vi "Format_Request.vi"(8 "error in (no error)":errorcluster, 10 "Request":T1(ring), 11 "Request in":refnum<class "Request.lvclass">) -> (0 "error out":errorcluster, 3 "Request out":refnum<class "Request.lvclass">)   [LabVIEW 2016, in "Request.lvclass"]
uses:
  Request.lvclass
  Request.lvclass/Request.ctl
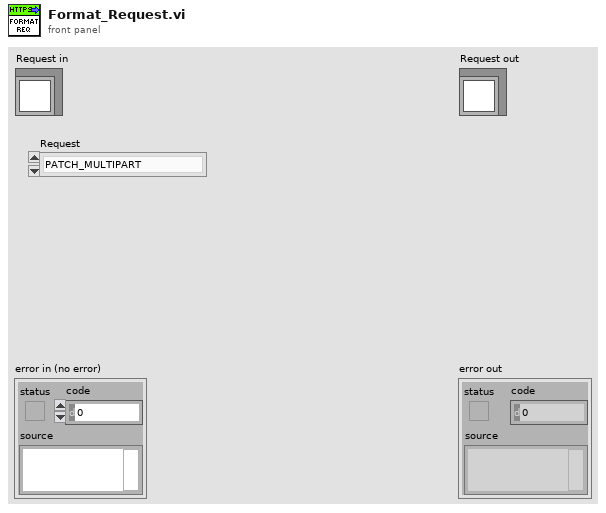
[diagram p1: front panel]
types:
  T1 = enum16{"PATCH_MULTIPART", "POST_MULTIPART", "PATCH", "DELETE", "HEAD", "PUT", "GET"}
  T2 = cluster{"Name":string, "Value":string, "File":path, "Filename":string, "MIME type":string}[]
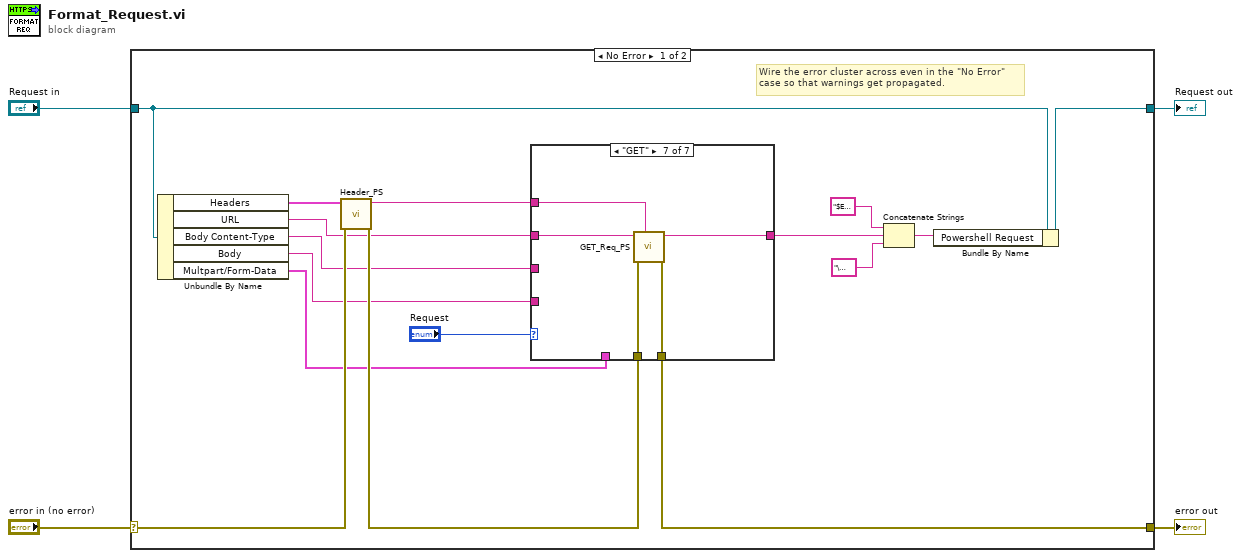
[diagram p0: block diagram]
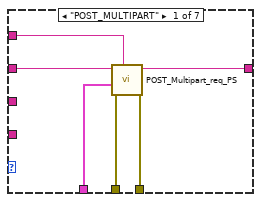
[diagram p2: hidden frame]
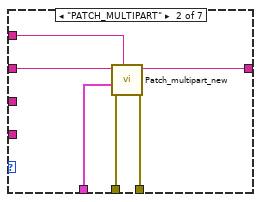
[diagram p3: hidden frame]
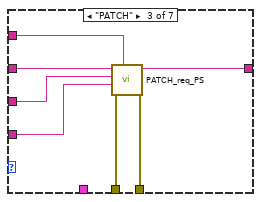
[diagram p4: hidden frame]
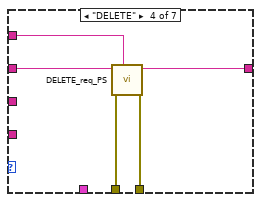
[diagram p5: hidden frame]
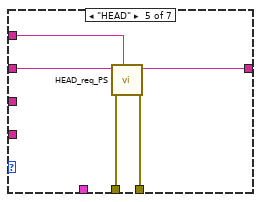
[diagram p6: hidden frame]
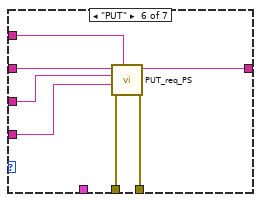
[diagram p7: hidden frame]
diagram:
  n1 = case shown="No Error" "error in (no error)" {
    selector: "error in (no error)" -> [w15 w63]
    tunnel: [w9 w63] -> w3
    tunnel: [w7 w62] -> w1
    tunnel: "Request in" -> [w8 w62]
    frame No Error {
      # "Wire the error cluster across even in the \"No Error\"\ncase so that warnings get propagated."
      n2 = Unbundle By Name(w8) -> ("Headers"=w14:cluster{"Name":string, "Value":string}[], "URL"=w13:string, "Body Content-Type"=w12:string, "Body"=w11:string, "Multpart/Form-Data"=w10:T2)
      n3 = call "Header_PS.vi"("error in"=w15, "Headers In"=w14) -> ("error out"=w16:errorcluster, "Headers_PS_Dict"=w17:string)  [unwired: 8 in]
      n4 = case shown="\"GET\"" "Request" {
        tunnel: w10 -> [w26 w27 _ _ _ _ _]
        tunnel: w13 -> [w23 w31 w39 w41 w47 w56 w58]
        tunnel: w16 -> [w25 w29 w38 w44 w49 w53 w59]
        tunnel: [w24 w28 w37 w43 w48 w52 w60] -> w9
        tunnel: w17 -> [w22 w32 w36 w40 w46 w51 w57]
        tunnel: [w21 w30 w33 w42 w45 w50 w61] -> w18
        tunnel: w12 -> [_ _ w34 _ _ w55 _]
        tunnel: w11 -> [_ _ w35 _ _ w54 _]
        frame "POST_MULTIPART" {
          n5 = call "POST_Multipart_req_PS.vi"("Headers"=w22, "error in"=w25, "Multpart/Form-Data"=w26, "URL"=w23) -> ("error out"=w24:errorcluster, "Multipart PATCH Request"=w21:string)  [unwired: 6 in]
        }
        frame "PATCH_MULTIPART" {
          n6 = call "Patch_multipart_new.vi"("Headers"=w32, "error in"=w29, "Multpart/Form-Data"=w27, "URL"=w31) -> ("error out"=w28:errorcluster, "Multipart PATCH Request"=w30:string)  [unwired: 6 in]
        }
        frame "PATCH" {
          n7 = call "PATCH_req_PS.vi"("Headers"=w36, "error in"=w38, "Body"=w35, "ContentType"=w34, "URL"=w39) -> ("error out"=w37:errorcluster, "PATCH Request"=w33:string)  [unwired: 5 in]
        }
        frame "DELETE" {
          n8 = call "DELETE_req_PS.vi"("Headers"=w40, "error in"=w44, "URL"=w41) -> ("error out"=w43:errorcluster, "DELETE Request"=w42:string)  [unwired: 7 in]
        }
        frame "HEAD" {
          n9 = call "HEAD_req_PS.vi"("Headers"=w46, "error in"=w49, "URL"=w47) -> ("error out"=w48:errorcluster, "HEAD Request"=w45:string)  [unwired: 7 in]
        }
        frame "PUT" {
          n10 = call "PUT_req_PS.vi"("Headers"=w51, "error in"=w53, "ContentType"=w54, "Body"=w55, "URL"=w56) -> ("error out"=w52:errorcluster, "PUT Request"=w50:string)  [unwired: 5 in]
        }
        frame "GET" {
          n11 = call "GET_Req_PS.vi"("Headers"=w57, "error in"=w59, "URL"=w58) -> ("error out"=w60:errorcluster, "GET Request"=w61:string)  [unwired: 7 in]
        }
      }
      n12 = Concatenate Strings("$ErrorActionPreference = \"SilentlyContinue\"\n" ("string"), w18, "\nWrite-Host \"StatusCode\"\nWrite-Host \"START\"\n$request.StatusCode\nWrite-Host \"END\"\nWrite-Host \"StatusDescription\"\nWrite-Host \"START\"\n$request.StatusDescription\nWrite-Host \"END\"\nWrite-Host \"Headers\"\nWrite-Host \"START\"\n$request.headers | convertto-json\nWrite-Host \"END\"\nWrite-Host \"Content\"\nWrite-Host \"START\"\n$request.content\nWrite-Host \"END\"\nWrite-Host \"Errors\"\nWrite-Host \"START\"\n$error\nWrite-Host \"END\"" ("string")) -> (w6:string)
      n13 = Bundle By Name(cluster=w8, "Powershell Request"=w6) -> (w7:refnum<class "Request.lvclass">)
    }
    frame Error {
    }
  }
  "error out" <- w3
  "Request out" <- w1
